vi "SSH Close.vi"(8 "Error In":errorcluster, 11 "SSH Session":refnum<k24>) -> (0 "Error Out":errorcluster)   [LabVIEW 2014, in "LMH-LINX.lvlib"]
uses:
  <vilib>/MakerHub/LINX/LMH-LINX.lvlib
  C:/Program Files (x86)/National Instruments/LabVIEW 2014/vi.lib/MakerHub/LINX/Resources/Renci.SshNet.dll
  Resources/Renci.SshNet.dll
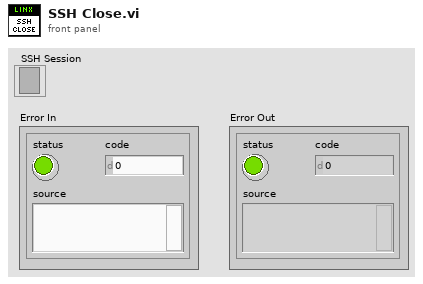
[diagram p1: front panel]
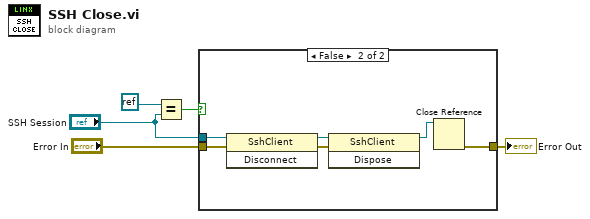
[diagram p0: block diagram]
diagram:
  n1 = Equal?(x=refnum<k0> refnum, y="SSH Session") -> (x = y?=w2:bool)
  n2 = case shown="False" w2 {
    tunnel: "Error In" -> [w6 w10]
    tunnel: [w6 w9] -> w4
    tunnel: "SSH Session" -> [_ w7]
    frame True {
    }
    frame False {
      n3 = invoke class="SshClient" method="Disconnect"(reference=w7, error in=w10) -> (reference out=w11:refnum<k24>, error out=w12:errorcluster)  [unwired: 1 in, 1 out]
      n4 = invoke class="SshClient" method="Dispose"(reference=w11, error in=w12) -> (reference out=w8:refnum<k24>)  [unwired: 1 in, 2 out]
      n5 = Close Reference(reference=w8) -> (error out=w9:errorcluster)  [unwired: 1 in]
    }
  }
  "Error Out" <- w4
